vi "ping.vi"(8 "error in (no error)":errorcluster, 11 "MB_TCP in":refnum<class "WebSocket Client CR.lvclass">) -> (0 "error out":errorcluster, 2 "Ping OK":bool, 3 "MB_TCP out":refnum<class "WebSocket Client CR.lvclass">)   [LabVIEW 2021, in "WebSockets.lvlib" / "WebSocket Client CR.lvclass"]
uses:
  WebSocket Client CR.lvclass
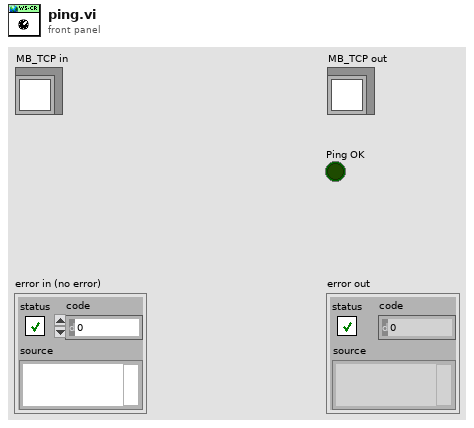
[diagram p1: front panel]
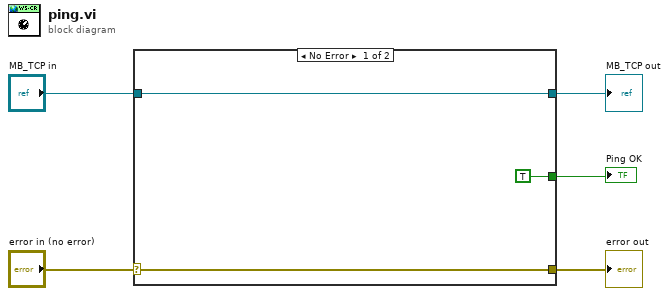
[diagram p0: block diagram]
diagram:
  n1 = case shown="No Error" "error in (no error)" {
    selector: "error in (no error)" -> [w7 w10]
    tunnel: [w7 w10] -> w4
    tunnel: [w8 w9] -> w2
    tunnel: "MB_TCP in" -> [w8 w9]
    tunnel: [TRUE ("Ping OK") _] -> w1
    frame No Error {
    }
    frame Error {
    }
  }
  "error out" <- w4
  "MB_TCP out" <- w2
  "Ping OK" <- w1
